vi "MGI Handle Show UI.vi"(8 "error in (no error)":errorcluster, 11 "MGI Error Reporter Dialog In":refnum<class "MGI Error Reporter Dialog.lvclass">) -> (0 "error out":errorcluster, 3 "MGI Error Reporter Dialog Out":refnum<class "MGI Error Reporter Dialog.lvclass">)   [LabVIEW 2020, in "MGI Error Reporter Dialog.lvclass"]
doc: "Handles showing the user interface for the error reporter, which is the Error Reporter daemon.\n\nAuthored by Shawn Walpole\nsupport@mooregoodideas.com\nwww.mooregoodideas.com\n\nCopyright (c) 2013, Moore Good Ideas, Inc.\n\nAll rights reserved.\n\nRedistribution and use in source and binary forms, with or without modification, are permitted provided that the following conditions are met:\n\n * Redistributions of source code must retain the above copyright notice, this list of conditions and the following disclaimer.\n * Redistributions in binary form must reproduce the above copyright notice, this list of conditions and the following disclaimer in the documentation and/or other materials provided with the distribution.\n * Neither the name of Moore Good Ideas, Inc. nor the names of its contributors may be used to endorse or promote products derived from this software without specific prior written permission.\n\nTHIS SOFTWARE IS PROVIDED BY THE COPYRIGHT HOLDERS AND CONTRIBUTORS \"AS IS\" AND ANY EXPRESS OR IMPLIED WARRANTIES, INCLUDING, BUT NOT LIMITED TO, THE IMPLIED WARRANTIES OF MERCHANTABILITY AND FITNESS FOR A PARTICULAR PURPOSE ARE DISCLAIMED. IN NO EVENT SHALL THE COPYRIGHT OWNER OR CONTRIBUTORS BE LIABLE FOR ANY DIRECT, INDIRECT, INCIDENTAL, SPECIAL, EXEMPLARY, OR CONSEQUENTIAL DAMAGES (INCLUDING, BUT NOT LIMITED TO, PROCUREMENT OF SUBSTITUTE GOODS OR SERVICES; LOSS OF USE, DATA, OR PROFITS; OR BUSINESS INTERRUPTION) HOWEVER CAUSED AND ON ANY THEORY OF LIABILITY, WHETHER IN CONTRACT, STRICT LIABILITY, OR TORT (INCLUDING NEGLIGENCE OR OTHERWISE) ARISING IN ANY WAY OUT OF THE USE OF THIS SOFTWARE, EVEN IF ADVISED OF THE POSSIBILITY OF SUCH DAMAGE."
uses:
  <userlib>/_MGI/Error Reporter/MGI Error Reporter Dialog/MGI Error Reporter Dialog.lvclass
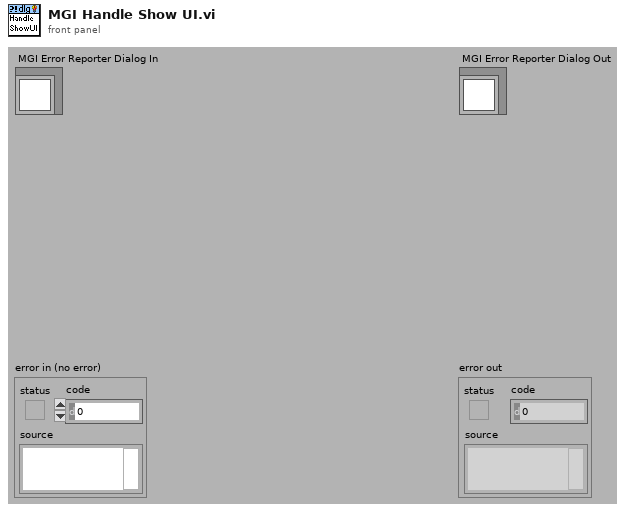
[diagram p1: front panel]
types:
  T1 = enum32{"Invalid", "Standard", "Closed", "Hidden", "Minimized", "Maximized"}
  T2 = typedef "MGI Error Reporter Dialog.lvclass/MGI Dialog UI Refs Cluster.ctl" = cluster{"LB Ref":refnum<vi>, "Details Ref":refnum<vi>, "Caller Ring Ref":refnum<vi>, "Message Ref":refnum<vi>, "Clear Btn Ref":refnum<vi>}
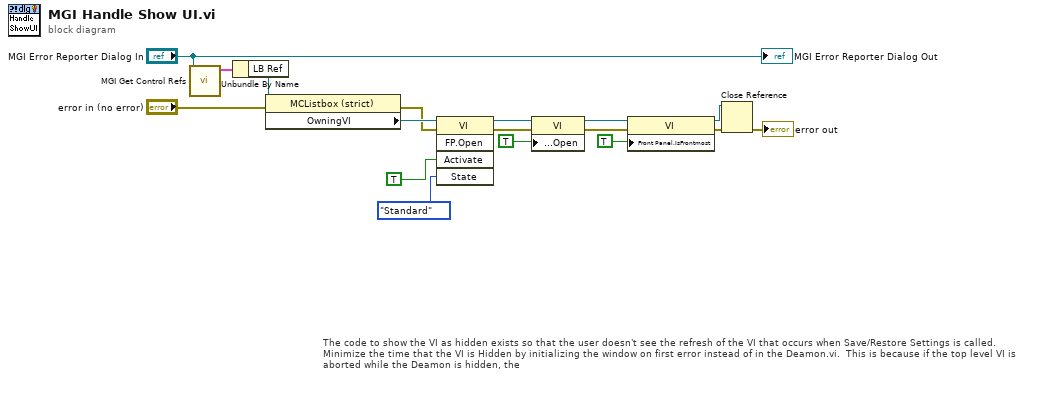
[diagram p0: block diagram]
diagram:
  # "The code to show the VI as hidden exists so that the user doesn't see the refresh of the VI that occurs when Save/Restore Settings is called.\nMinimize the time that the VI is Hidden by initializing the window on first error instead of in the Deamon.vi.  This is because if the top level VI is aborted while the Deamon is hidden, the"
  n1 = call <userlib>:"MGI Get Control Refs.vi"("MGI Error Dialog.lvclass"="MGI Error Reporter Dialog In") -> ("Refs"=w15:T2)  [unwired: 10 out]
  n2 = Unbundle By Name(w15) -> ("LB Ref"=w14:refnum<vi>)
  n3 = property class="MCListbox (strict)"(reference=w14, error in="error in (no error)") -> (error out=w1:errorcluster, "OwningVI"=w2:refnum<vi>)  [unwired: 1 out]
  n4 = invoke class="VI" method="FP.Open"(reference=w2, error in=w1, "Activate"=TRUE ("Front Panel Window:Open"), "State"=T1."Standard") -> (reference out=w9:refnum<vi>, error out=w7:errorcluster)  [unwired: 1 in, 3 out]
  n5 = property class="VI"(reference=w9, error in=w7, "Front Panel.Open"=TRUE ("Front Panel Window:Open")) -> (reference out=w11:refnum<vi>, error out=w10:errorcluster)
  n6 = property class="VI"(reference=w11, error in=w10, "Front Panel.IsFrontmost"=TRUE ("Front Panel Window:Is Frontmost")) -> (reference out=w5:refnum<vi>, error out=w4:errorcluster)
  n7 = Close Reference(reference=w5, error in (no error)=w4) -> (error out=→"error out":errorcluster)
  "MGI Error Reporter Dialog Out" <- "MGI Error Reporter Dialog In"
